vi "Configure Frequency Period.vi"(4 "Auto Timeout (F: Disable)":bool, 5 "Voltage Range (10: 10 V)":dbl(ring)=10.0 items=["0.1"=0.1, "1"=1.0, "10"=10.0, "100"=100.0, "1000"=1000.0], 6 "Auto Voltage Range (1: Enable)":i32(ring)=1 items=["Disable", "Enable", "Once"], 7 "AC Bandwidth (20: 20 Hz)":dbl(ring)=20.0 items=["3"=3.0, "20"=20.0, "200"=200.0], 8 "error in (no error)":errorcluster, 9 "Aperture Time (0.1: 0.1 s)":dbl(ring)=0.1 items=["0.01"=0.01, "0.1"=0.1, "1"=1.0], 10 "Frequency Period (0: Frequency)":i32(ring) items=["Frequency", "Period"], 11 "VISA resource name":refnum<visa-resource-name>) -> (0 "error out":errorcluster, 3 "VISA resource name out":refnum<visa-resource-name>)   [LabVIEW 2020, in "Agilent 3446X Series.lvlib"]
doc: "Configures frequency and period measurements."
uses:
  <instrlib>/Agilent 3446X Series/Agilent 3446X Series.lvlib
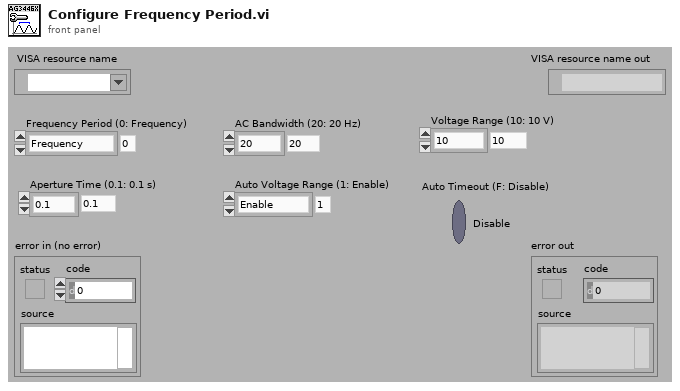
[diagram p1: front panel]
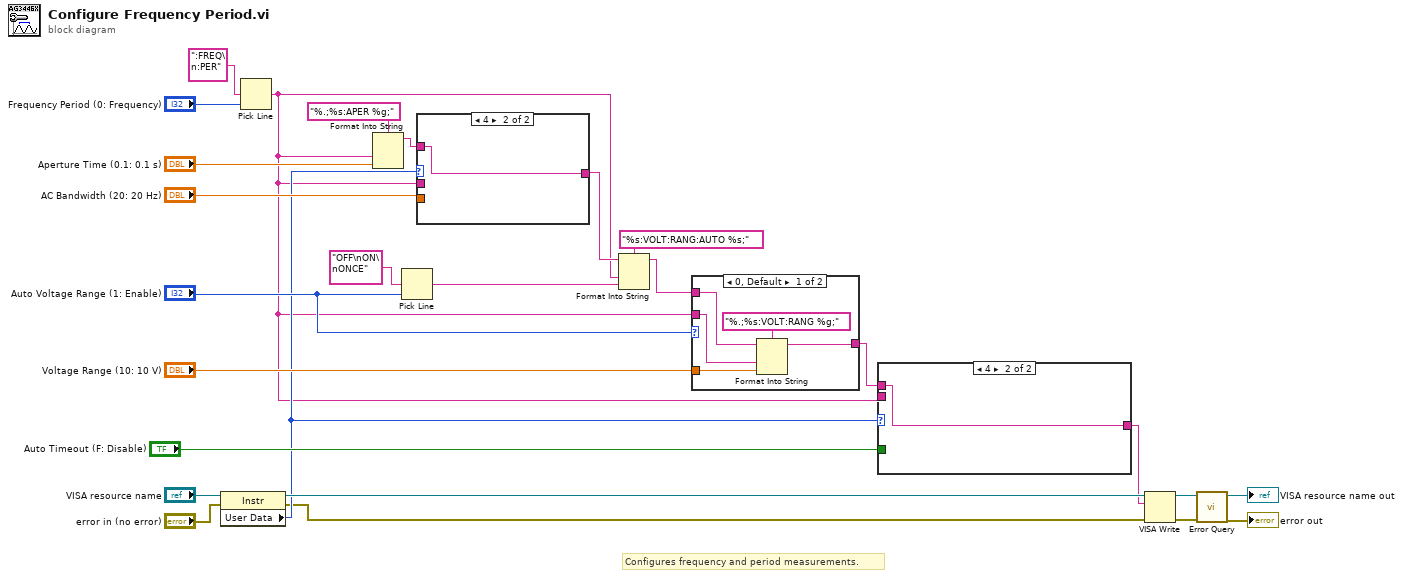
[diagram p0: block diagram]
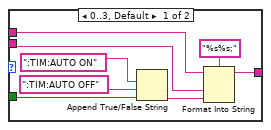
[diagram p2: hidden frame]
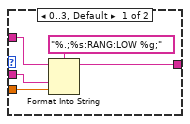
[diagram p3: hidden frame]
diagram:
  # "Configures frequency and period measurements."
  n1 = property class="Instr"(reference="VISA resource name", error in="error in (no error)") -> (reference out=w19:refnum<visa-resource-name>, error out=w2:errorcluster, "User Data"=w4:u32)
  n2 = Pick Line(multi-line string=":FREQ\n:PER", line index="Frequency Period (0: Frequency)") -> (output string=w1:string)  [unwired: 1 out]
  n3 = Format Into String(format string="%.;%s:APER %g;", w1, "Aperture Time (0.1: 0.1 s)") -> (resulting string=w17:string)  [unwired: 2 in, 1 out]
  n4 = Pick Line(multi-line string="OFF\nON\nONCE", line index="Auto Voltage Range (1: Enable)") -> (output string=w13:string)  [unwired: 1 out]
  n5 = case shown="4" w4 {
    tunnel: w17 -> [w31 w32]
    tunnel: [w29 w32] -> w15
    tunnel: w1 -> [w28 _]
    tunnel: "AC Bandwidth (20: 20 Hz)" -> [w27 _]
    frame 0..3, Default {
      n6 = Format Into String(format string="%.;%s:RANG:LOW %g;", initial string=w31, w28, w27) -> (resulting string=w29:string)  [unwired: 1 in, 1 out]
    }
    frame 4 {
    }
  }
  n7 = Format Into String(format string="%s:VOLT:RANG:AUTO %s;", initial string=w15, w1, w13) -> (resulting string=w12:string)  [unwired: 1 in, 1 out]
  n8 = case shown="0, Default" "Auto Voltage Range (1: Enable)" {
    tunnel: "Voltage Range (10: 10 V)" -> [w36 _]
    tunnel: w1 -> [w35 _]
    tunnel: w12 -> [w34 w38]
    tunnel: [w33 w38] -> w11
    frame 0, Default {
      n9 = Format Into String(format string="%.;%s:VOLT:RANG %g;", initial string=w34, w35, w36) -> (resulting string=w33:string)  [unwired: 1 in, 1 out]
    }
    frame 1, 2 {
    }
  }
  n10 = case shown="4" w4 {
    tunnel: w11 -> [w42 w47]
    tunnel: "Auto Timeout (F: Disable)" -> [w41 _]
    tunnel: [w40 w47] -> w5
    tunnel: w1 -> [w39 _]
    frame 0..3, Default {
      n11 = Append True/False String(1:w41, 2:":TIM:AUTO OFF" ("false string"), 3:":TIM:AUTO ON" ("true string")) -> (0:w43:string)  [unwired: 1 in]
      n12 = Format Into String(format string="%s%s;", initial string=w42, w39, w43) -> (resulting string=w40:string)  [unwired: 1 in, 1 out]
    }
    frame 4 {
    }
  }
  n13 = VISA Write(VISA resource name=w19, write buffer=w5, error in (no error)=w2) -> (VISA resource name out=w24:refnum<visa-resource-name>, error out=w23:errorcluster)  [unwired: 1 out]
  n14 = call <instrlib>:"Error Query.vi"("error in (no error)"=w23, "VISA resource name"=w24) -> ("error out"=→"error out":errorcluster, "VISA resource name out"=→"VISA resource name out":refnum<visa-resource-name>)  [unwired: 8 out]
